vi "Init.vi"(8 "error in (no error)":errorcluster, 11 "PDE_Wave_2D":refnum<class "NI_PDE_Wave_2D.lvclass">) -> (0 "error out":errorcluster, 3 "initialized PDE_Wave_2D":refnum<class "NI_PDE_Wave_2D.lvclass">)   [LabVIEW 2020, in "NI_PDE.lvlib" / "NI_PDE_Wave_2D.lvclass"]
uses:
  <vilib>/gmath/pde.llb/PDEClass/PDE_Wave_2D/NI_PDE_Wave_2D.lvclass
  <vilib>/gmath/pde.llb/PDEClass/Class Type.ctl
  <vilib>/gmath/pde.llb/PDEClass/PDE_2ndOrder_ConstPara/NI_PDE_2ndOrder_ConstPara.lvclass
  <vilib>/gmath/pde.llb/PDEClass/NI_PDE.lvclass
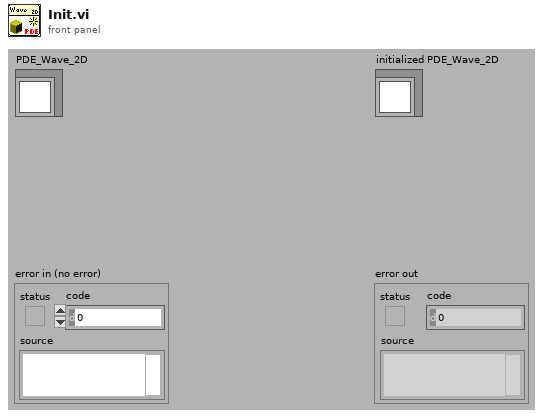
[diagram p1: front panel]
types:
  T1 = typedef "NI_PDE.lvlib/NI_PDE.lvclass/Class Type.ctl" = i32
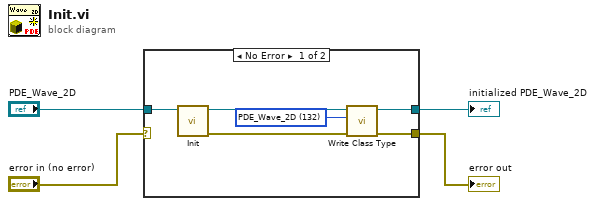
[diagram p0: block diagram]
diagram:
  n1 = case shown="No Error" "error in (no error)" {
    selector: "error in (no error)" -> [_ w11]
    tunnel: [w8 w11] -> w4
    tunnel: [w9 w12] -> w3
    tunnel: "PDE_Wave_2D" -> [w7 w12]
    frame No Error {
      w10 = T1 132 items=["PDE"=0, "PDE_2ndOrder_ConstPara"=100, "PDE_Helmholtz_2D"=112, "PDE_Heat_1D"=121, "PDE_Heat_2D"=122, "PDE_Wave_1D"=131, "PDE_Wave_2D"=132] ("PDE class type")
      n2 = call-parent "Init.vi"("PDE_2ndOrder_ConstPara"=w7) -> ("error out"=w5:errorcluster, "initialized PDE_2ndOrder_ConstPara"=w6:refnum<class "NI_PDE_Wave_2D.lvclass">)  [unwired: 1 in, 8 out]
      n3 = call-dynamic "Write Class Type.vi"("error in (no error)"=w5, "PDE class type"=w10, "PDE.lvclass in"=w6) -> ("error out"=w8:errorcluster, "PDE.lvclass out"=w9:refnum<class "NI_PDE_Wave_2D.lvclass">)  [unwired: 7 out]
    }
    frame Error {
    }
  }
  "initialized PDE_Wave_2D" <- w3
  "error out" <- w4
